vi "Initialize PID Controller Channel Browsers.vi"(6 "Use External Setpoint":bool, 7 "Output":refnum<k24>(container), 8 "error in (no error)":errorcluster, 9 "Feedback":refnum<k24>(container), 10 "Setpoint in":refnum<k24>(container) caption="Setpoint", 11 "Item Ref in":T2 format="%.0x") -> (0 "error out":errorcluster, 2 "Refs":T1, 3 "Item Ref out":T2 format="%.0x")   [LabVIEW 2015, in "Control Addon System Explorer.lvlib"]
uses:
  Control Addon System Explorer.lvlib
  NationalInstruments.VeriStand.SystemStorageUI
  <vilib>/NI Veristand/Custom Device API/Custom Device Item Ref.ctl
  Types/PID Controller Channel Browser Refs.ctl
  <vilib>/NI Veristand/UI Controls/Single Node Browser/Net Event Data.ctl
  <vilib>/NI Veristand/UI Controls/Single Node Browser/Net Event.ctl
  Shared/Constants.vi
  Shared/Control Addon Shared.lvlib
  <vilib>/NI Veristand/UI Controls/Single Node Browser/NI_VS UI Single Node Browser.lvlib
  <vilib>/NI VeriStand/Custom Device API/Custom Device API.lvlib
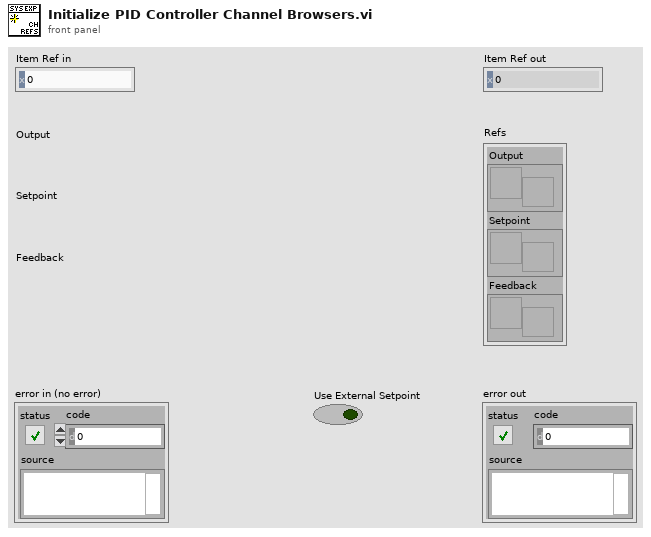
[diagram p1: front panel]
types:
  T1 = typedef "Control Addon System Explorer.lvlib/PID Controller Channel Browser Refs.ctl" = cluster{"Output":refnum<user-event>, "Setpoint":refnum<user-event>, "Feedback":refnum<user-event>}
  T2 = typedef "Custom Device API.lvlib/Custom Device Item Ref.ctl" = u64
  T3 = typedef "NI_VS UI Single Node Browser.lvlib/Single Node Browser Ref.ctl" = refnum<k24>
  T4 = typedef "NI_VS UI Single Node Browser.lvlib/Callback Type.ctl" = cluster{"Net Callbacks":refnum<k27>[], "Event":refnum<user-event>}
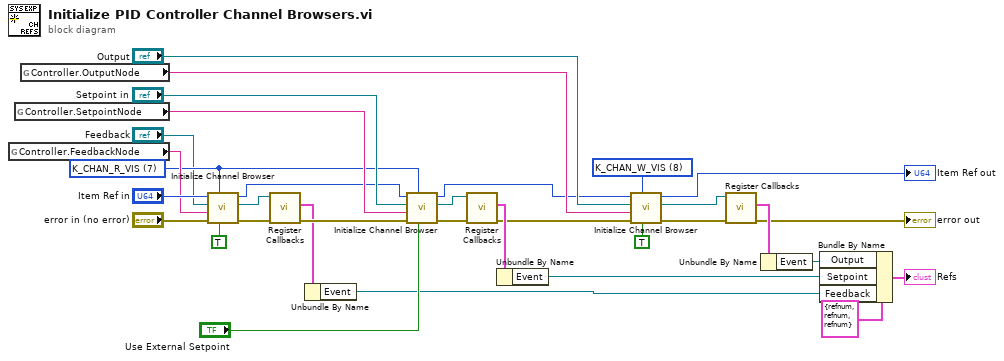
[diagram p0: block diagram]
diagram:
  w13 = u8 7 items=["K_CHAN_R", "K_CHAN_W", "K_CHAN_RW", "K_CHAN_VOLT", "K_CHAN_FAULT", "K_ALL", "K_CUSTOM", "K_CHAN_R_VIS", "K_CHAN_W_VIS", "K_CHAN_RW_VIS", "K_CHAN_VOLT_VIS", "K_CHAN_FAULT_VIS"] ("DisplayFilter")
  w12 = u8 8 items=["K_CHAN_R", "K_CHAN_W", "K_CHAN_RW", "K_CHAN_VOLT", "K_CHAN_FAULT", "K_ALL", "K_CUSTOM", "K_CHAN_R_VIS", "K_CHAN_W_VIS", "K_CHAN_RW_VIS", "K_CHAN_VOLT_VIS", "K_CHAN_FAULT_VIS"] ("DisplayFilter")
  n1 = global read "Constants.vi" "Controller.FeedbackNode"() -> (w16:string)
  n2 = global read "Constants.vi" "Controller.SetpointNode"() -> (w32:string)
  n3 = global read "Constants.vi" "Controller.OutputNode"() -> (w17:string)
  n4 = call "Initialize Channel Browser.vi"("Use Channel?"=TRUE, "DisplayFilter"=w13, "error in (no error)"="error in (no error)", "NodeName"=w16, "Browser Ref"="Feedback", "Item Ref in"="Item Ref in") -> ("error out"=w21:errorcluster, "Browser Ref"=w23:T3, "Item Ref out"=w2:T2)  [unwired: 3 in]
  n5 = call <vilib>:"Register Callbacks.vi"("error in (no error)"=w21, "Single Node Browser"=w23) -> ("error out"=w22:errorcluster, "Callbacks"=w20:T4)  [unwired: 7 in, 1 out]
  n6 = Unbundle By Name(w20) -> ("Event"=w3:refnum<user-event>)
  n7 = call "Initialize Channel Browser.vi"("Use Channel?"="Use External Setpoint", "DisplayFilter"=w13, "error in (no error)"=w22, "NodeName"=w32, "Browser Ref"="Setpoint in", "Item Ref in"=w2) -> ("error out"=w7:errorcluster, "Browser Ref"=w25:T3, "Item Ref out"=w8:T2)  [unwired: 3 in]
  n8 = call <vilib>:"Register Callbacks.vi"("error in (no error)"=w7, "Single Node Browser"=w25) -> ("error out"=w24:errorcluster, "Callbacks"=w26:T4)  [unwired: 7 in, 1 out]
  n9 = Unbundle By Name(w26) -> ("Event"=w4:refnum<user-event>)
  n10 = call "Initialize Channel Browser.vi"("Use Channel?"=TRUE, "DisplayFilter"=w12, "error in (no error)"=w24, "NodeName"=w17, "Browser Ref"="Output", "Item Ref in"=w8) -> ("error out"=w28:errorcluster, "Browser Ref"=w27:T3, "Item Ref out"=→"Item Ref out":T2)  [unwired: 3 in]
  n11 = call <vilib>:"Register Callbacks.vi"("error in (no error)"=w28, "Single Node Browser"=w27) -> ("error out"=→"error out":errorcluster, "Callbacks"=w30:T4)  [unwired: 7 in, 1 out]
  n12 = Unbundle By Name(w30) -> ("Event"=w5:refnum<user-event>)
  n13 = Bundle By Name(cluster=T1 {"Output"=refnum, "Setpoint"=refnum, "Feedback"=refnum} ("Refs"), "Output"=w5, "Setpoint"=w4, "Feedback"=w3) -> (→"Refs":T1)
